vi "Obtain Queue.vi"(8 "error in (no error)":errorcluster, 11 "Helper Loop in":refnum<class "Helper Loop.lvclass">) -> (0 "error out":errorcluster, 3 "Helper Loop out":refnum<class "Helper Loop.lvclass">)   [LabVIEW 2024, in "Helper Loop.lvlib" / "Helper Loop.lvclass"]
uses:
  Helper Loop.lvclass
  Helper Loop.lvclass/Helper Loop.ctl
  messages.ctl
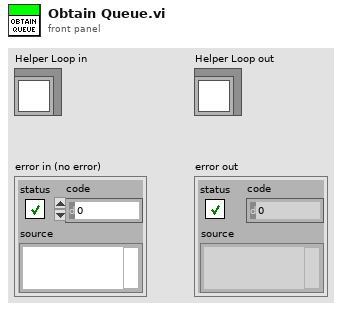
[diagram p1: front panel]
types:
  T1 = typedef "Helper Loop.lvlib/Helper Loop.lvclass/messages.ctl" = enum16{"start polling", "stop polling", "poll", "exit"}
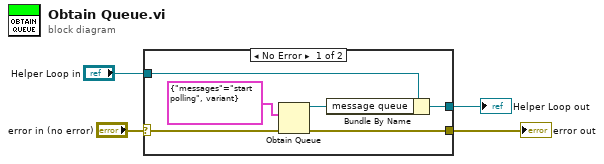
[diagram p0: block diagram]
diagram:
  n1 = case shown="No Error" "error in (no error)" {
    selector: "error in (no error)" -> [w8 w12]
    tunnel: [w7 w12] -> w3
    tunnel: [w6 w11] -> w1
    tunnel: "Helper Loop in" -> [w9 w11]
    frame No Error {
      n2 = Obtain Queue(element data type=cluster{"messages":T1, variant} {"messages"=enum."start polling", variant}, error in (no error)=w8) -> (queue out=w5:refnum<queue>, error out=w7:errorcluster)  [unwired: 3 in, 1 out]
      n3 = Bundle By Name(cluster=w9, "message queue"=w5) -> (w6:refnum<class "Helper Loop.lvclass">)
    }
    frame Error {
    }
  }
  "error out" <- w3
  "Helper Loop out" <- w1
